vi "SetupListener.vi"(0 "Socket Listener in":refnum<class "Socket Communication.lvclass">, 5 "error in (no error)":errorcluster) -> (14 "Socket Listener out":refnum<class "Socket Communication.lvclass">, 19 "error out":errorcluster)   [LabVIEW 2019, in "Socket Communication.lvclass"]
uses:
  Socket Communication.lvclass
  Socket Communication.lvclass/Socket Communication.ctl
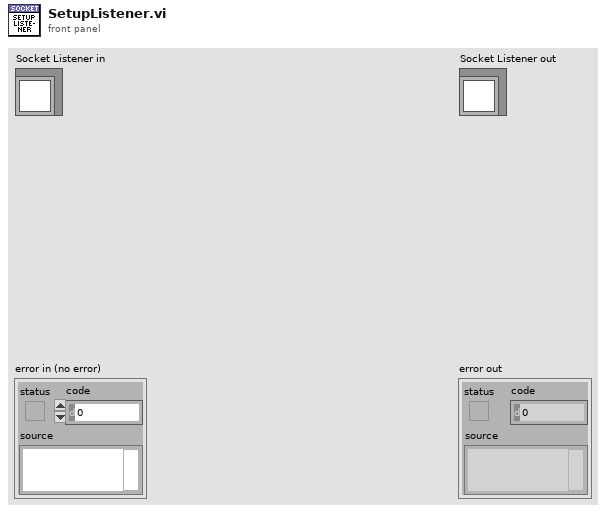
[diagram p1: front panel]
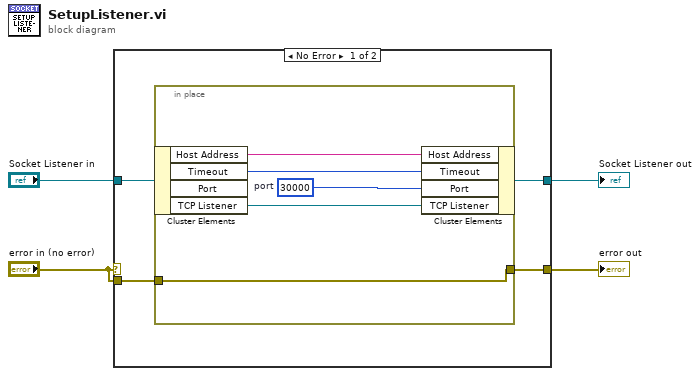
[diagram p0: block diagram]
diagram:
  n1 = case shown="No Error" "error in (no error)" {
    selector: "error in (no error)" -> [_ w14]
    tunnel: [w7 w15] -> w3
    tunnel: "Socket Listener in" -> [w8 w15]
    tunnel: [w5 w14] -> w2
    tunnel: "error in (no error)" -> [w6 _]
    frame No Error {
      n2 = in-place {
        in-place-border: w6 -> [w9]
        in-place-border: [w9] -> w5
        w13 = u16 30000  # port
        n3 = in-place-cluster #1(w8) -> ("Host Address"=w12:string, "Timeout"=w11:i32, "TCP Listener"=w10:refnum<k5>)  [unwired: 1 out]
        n4 = in-place-cluster #1("Host Address"=w12, "Timeout"=w11, "Port"=w13, "TCP Listener"=w10) -> (w7:refnum<class "Socket Communication.lvclass">)
      }
    }
    frame Error {
    }
  }
  "error out" <- w2
  "Socket Listener out" <- w3
